vi "DetectTransition(HtoL).vi"(11 "InputSignal":bool) -> (3 "FallingFront":bool)   [LabVIEW 2013]
doc: "Generate a pulse at the output when the input signal commutate from high to low"
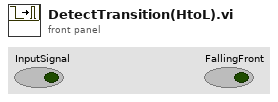
[diagram p1: front panel]
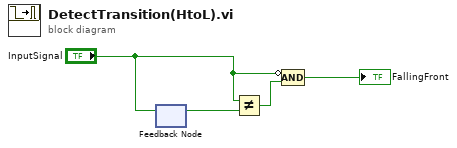
[diagram p0: block diagram]
diagram:
  n1 = feedback #1() -> (w4:bool)  [unwired: 1 in]
  n2 = feedback-in #1("InputSignal") -> ()
  n3 = Not Equal?(x="InputSignal", y=w4) -> (x != y?=w1:bool)
  n4 = Compound Arithmetic op=AND(invert "InputSignal", w1) -> (→"FallingFront":bool)
